vi "Save Sequence.vi"(8 "error in (no error)":errorcluster, 10 "Browse start path":path, 11 "Uncompiled sequence in":T1[](array[typedef])) -> (0 "error out":errorcluster)   [LabVIEW 2020, in "Sequencer.lvlib"]
doc: "Save the uncompiled sequence to a sequence file."
uses:
  Sequencer.lvlib
  Controls/Ctl_SequenceElement.ctl
  Controls/Ctl_SequenceControlElement.ctl
  PPL/HDH.Actor Framework.Core.Msg.lvlibp/Flex Msg/Controls/Ctl_Control Element.ctl
  PPL/HDH.Actor Framework.Core.Msg.lvlibp
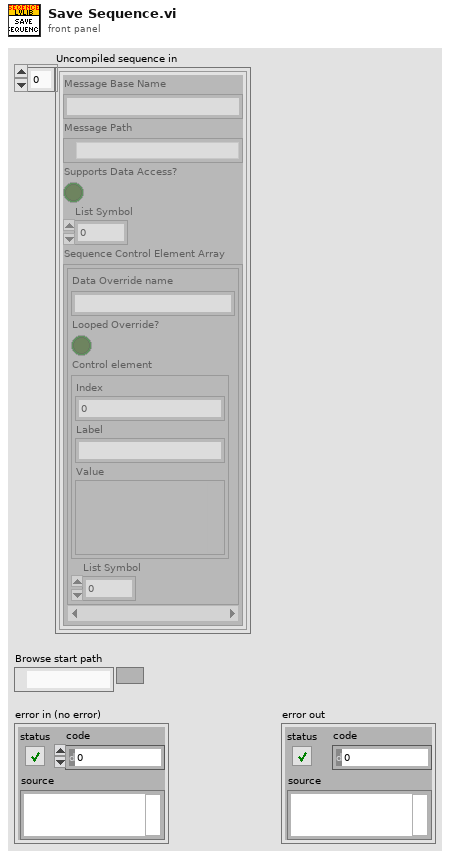
[diagram p1: front panel]
types:
  T1 = typedef "Sequencer.lvlib/Ctl_SequenceElement.ctl" = cluster{"Message Base Name":string, "Message Path":path, "Supports Data Access?":bool, "List Symbol":i32, "Sequence Control Element Array":T2[]}
  T2 = typedef "Sequencer.lvlib/Ctl_SequenceControlElement.ctl" = cluster{"Data Override name":string, "Looped Override?":bool, "Control element":T3, "List Symbol":i32}
  T3 = typedef "HDH.Actor Framework.Core.Msg.lvlibp/Ctl_Control Element.ctl" = cluster{"Index":i32, "Label":string, "Value":variant}
  T4 = enum16{"open", "replace", "create", "open or create", "replace or create", "replace or create with confirmation"}
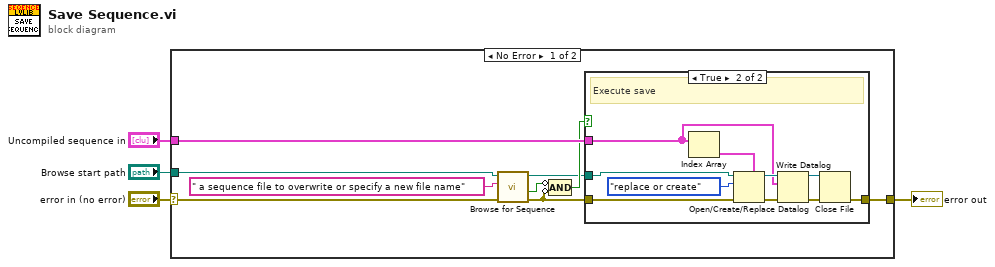
[diagram p0: block diagram]
diagram:
  n1 = case shown="No Error" "error in (no error)" {
    selector: "error in (no error)" -> [w6 w25]
    tunnel: [w13 w25] -> w4
    tunnel: "Uncompiled sequence in" -> [w12 _]
    tunnel: "Browse start path" -> [w10 _]
    frame No Error {
      n2 = call "Browse for Sequence.vi"("error in (no error)"=w6, "Caption (Browse for/Select concatenated)"=" a sequence file to overwrite or specify a new file name" ("prompt"), "Browse start path"=w10) -> ("error out"=w5:errorcluster, "Cancelled?"=w8:bool, "File Path out"=w9:path)  [unwired: 6 in]
      n3 = Compound Arithmetic op=AND(invert w8, invert w5) -> (w11:bool)
      n4 = case shown="True" w11 {
        tunnel: [w14 w15] -> w13
        tunnel: w5 -> [w14 w22]
        tunnel: w12 -> [_ w19]
        tunnel: w9 -> [_ w24]
        frame False {
          # "Cancelled or error"
        }
        frame True {
          # "Execute save"
          n5 = Index Array(array=w19) -> (element=w21:T1)  [unwired: 1 in]
          n6 = Open/Create/Replace Datalog(5:w21, 8:w22, 10:T4."replace or create" ("operation (0:open)"), 11:w24) -> (0:w18:errorcluster, 3:w20:refnum<k1>)  [unwired: 2 in, 1 out]
          n7 = Write Datalog(4:w18, 6:w19, 7:w20) -> (0:w16:errorcluster, 3:w17:refnum<k1>)
          n8 = Close File(refnum=w17, error in=w16) -> (error out=w15:errorcluster)  [unwired: 1 out]
        }
      }
    }
    frame Error {
    }
  }
  "error out" <- w4
